vi "GOTOxyz.vi"(6 "reset":bool, 7 "error in (no error)":errorcluster, 9 "Y":dbl format="%#_13g", 10 "X":dbl format="%#_13g") -> (0 "error out":errorcluster)   [LabVIEW 2018]
uses:
  <vilib>/Platform/TimedLoop/XDataNode/timing_clust.ctl
  <vilib>/Platform/TimedLoop/XDataNode/nitl_modes.ctl
  <vilib>/Platform/TimedLoop/XDataNode/wakeup.ctl
  <vilib>/platform/TimedLoop/XDataNode/XDataNode.xnode
  <vilib>/Platform/TimedLoop/XDataNode/XDNodeRunTimeDep.lvlib
  <vilib>/ptbypt/NI_PtbyPt.lvlib
panel:
  out "x*y":dbl
  out "theta":dbl
  in  "Z":dbl format="%#_13g"
  out "T1":dbl
  out "Waveform Chart":dbl(graph)
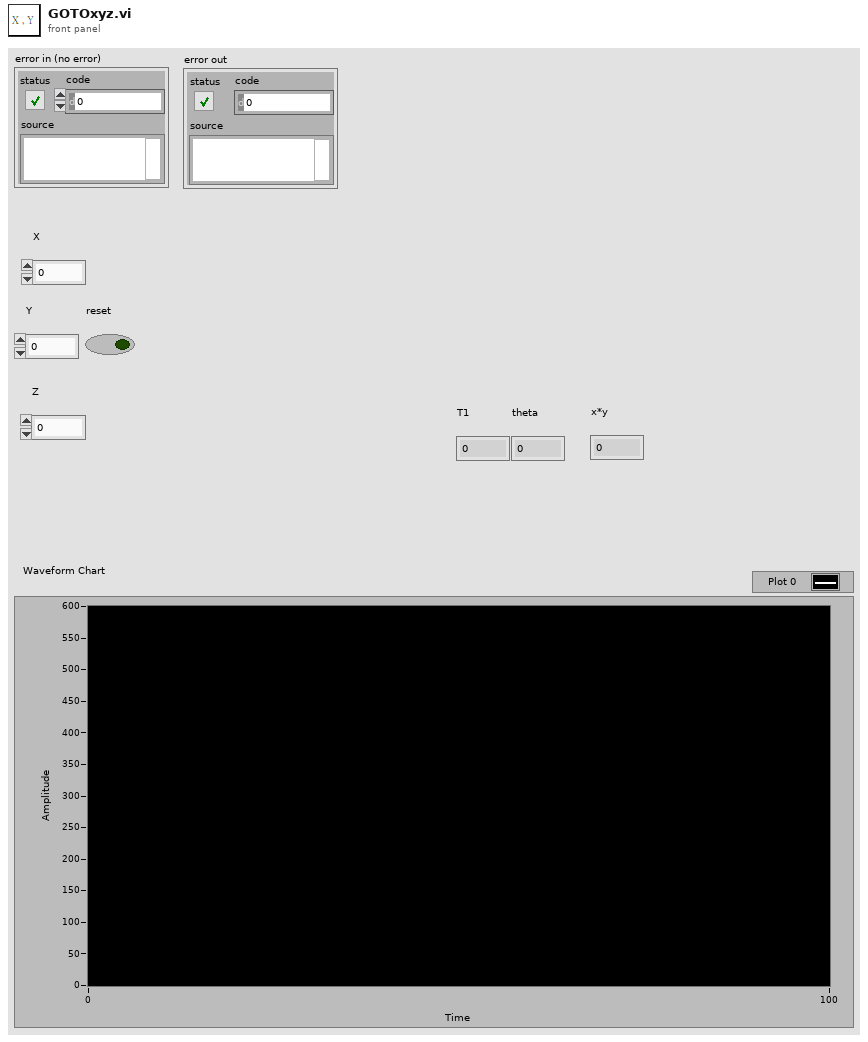
[diagram p1: front panel]
types:
  T1 = typedef "XDNodeRunTimeDep.lvlib/timing_clust.ctl" = cluster{"Expected End [f-1]":u64, "Actual End [f-1]":u64, "Finished Late? [f-1]":bool, "Expected End [i-1]":u64, "Actual End [i-1]":u64, "Finished Late? [i-1]":bool, "Expected Start [i]":u64, "Actual Start [i]":u64, "Expected Start [f]":u64, "Actual Start [f]":u64, "Source Name":string, "Structure Name":string, "Period":i64, "Deadline":i64, "Offset":i64, "Start":i64, "Priority":i32, "Timeout":i32, "Mode":T2, "Wakeup Reason":T3, "Error":errorcluster, "Source Type":string, "Secondary Source Type":string, "Global End Time":u64, "Global Start Time":u64, "Frame Duration":u64, "Iteration Duration":u64, "Assigned CPU":i32, "I/O Scan Engine Mode":u32}
  T2 = typedef "XDNodeRunTimeDep.lvlib/nitl_modes.ctl" = enum32{"No Change", "Process missed periods, maintain original phase", "Discard missed periods, maintain original phase", "Process missed periods, ignore original phase", "Discard missed periods, ignore original phase"}
  T3 = typedef "XDNodeRunTimeDep.lvlib/wakeup.ctl" = enum32{"Normal", "Aborted", "Asynchronous wakeup", "Timing source error", "Timed loop error", "Timeout"}
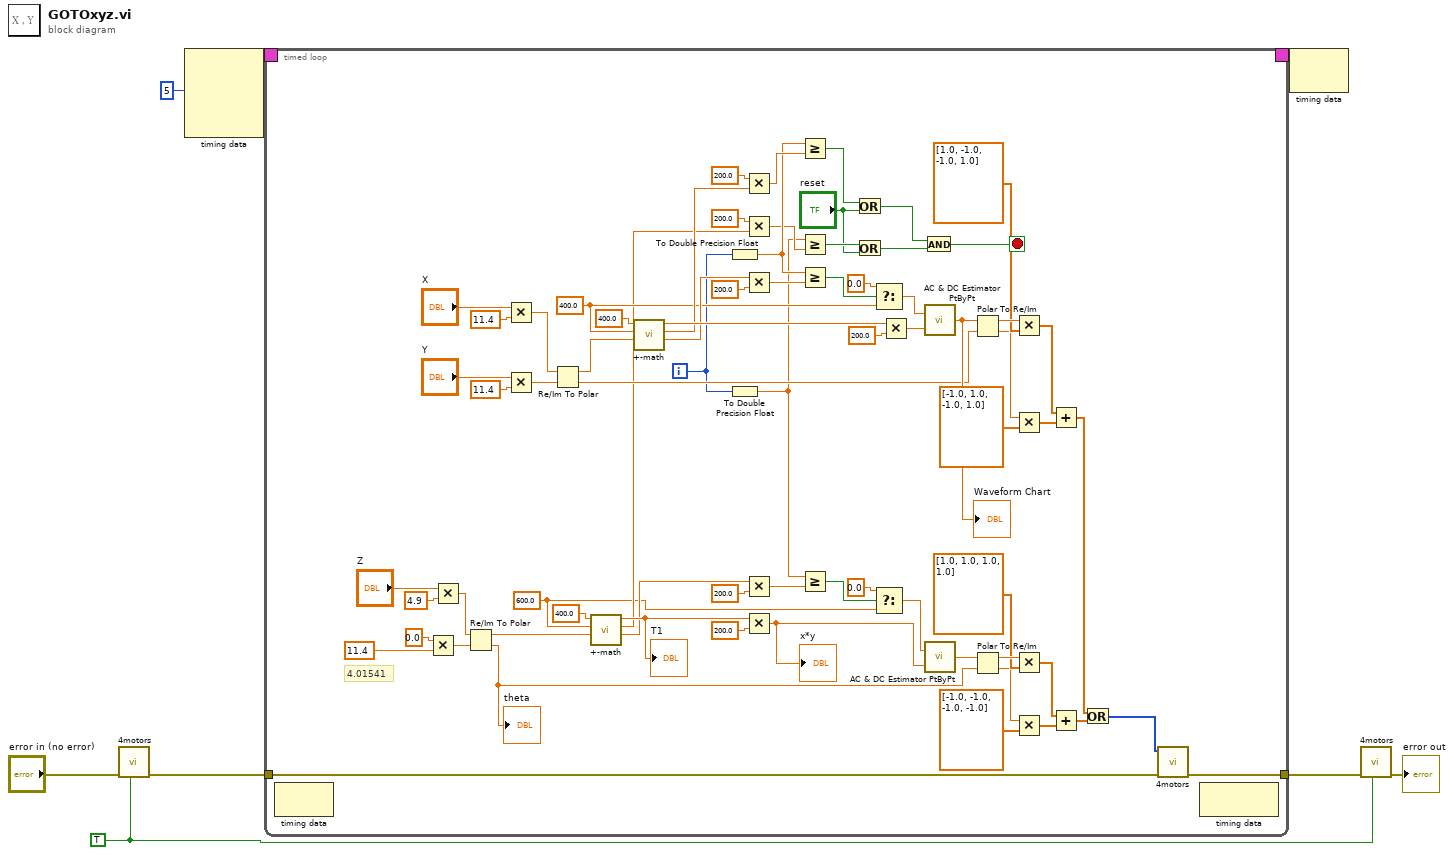
[diagram p0: block diagram]
diagram:
  w3 = TRUE ("Reset")
  n1 = call "4motors.vi"("Reset"=w3, "error in (no error)"="error in (no error)") -> ("error out"=w4:errorcluster)  [unwired: 8 in, 1 out]
  n2 = node-c288(i64 5 ("Period")) -> (w8:T1)  [unwired: 3 in]
  n3 = timed-loop {
    timing: w8 -> [_]
    timing-out: [_] -> w7
    tunnel: [w51] -> w5
    tunnel: w4 -> [w49]
    i -> [w10]
    stop <- w12 stop-if-true
    w18 = 600.0 ("VMAX")
    w50 = 400.0 ("VMAX")
    # "4.01541"
    n4 = node-c288() -> ()  [unwired: 1 in, 1 out]
    n5 = Multiply(x=0.0 ("Y"), y=11.4) -> (x*y=w24:dbl)
    n6 = Multiply(x="Z", y=4.9) -> (x*y=w27:dbl)
    n7 = Re/Im To Polar(2:w24, 3:w27) -> (0:w36:dbl, 1:w38:dbl)
    "theta" <- w36
    n8 = Multiply(x="X", y=11.4) -> (x*y=w60:dbl)
    n9 = Multiply(x="Y", y=11.4) -> (x*y=w57:dbl)
    n10 = Re/Im To Polar(2:w57, 3:w60) -> (0:w69:dbl, 1:w71:dbl)
    n11 = call "+-math.vi"("S"=w38, "VMAX"=w18, "ACC"=400.0) -> ("T2"=w43:dbl, "T3"=w23:dbl, "T1"=w46:dbl)  [unwired: 6 in]
    "T1" <- w46
    n12 = call "+-math.vi"("S"=w71, "VMAX"=w50, "ACC"=400.0) -> ("T2"=w76:dbl, "T3"=w56:dbl, "T1"=w79:dbl)  [unwired: 6 in]
    n13 = To Double Precision Float(number=w10) -> (double precision float=w48:dbl)
    n14 = To Double Precision Float(number=w10) -> (double precision float=w17:dbl)
    n15 = Multiply(x=200.0, y=w56) -> (x*y=w54:dbl)
    n16 = Multiply(x=200.0, y=w23) -> (x*y=w21:dbl)
    n17 = Multiply(x=w76, y=200.0) -> (x*y=w74:dbl)
    n18 = Multiply(x=w43, y=200.0) -> (x*y=w41:dbl)
    n19 = Multiply(x=w46, y=200.0) -> (x*y=w44:dbl)
    "x*y" <- w44
    n20 = Greater Or Equal?(x=w48, y=w54) -> (x >= y?=w53:bool)
    n21 = Greater Or Equal?(x=w17, y=w21) -> (x >= y?=w20:bool)
    n22 = Greater Or Equal?(x=w48, y=w74) -> (x >= y?=w52:bool)
    n23 = Greater Or Equal?(x=w17, y=w41) -> (x >= y?=w19:bool)
    n24 = Or(x=w53, y="reset") -> (x .or. y?=w13:bool)
    n25 = Or(x=w20, y="reset") -> (x .or. y?=w14:bool)
    n26 = Select(t=0.0, s=w52, f=w50) -> (s? t:f=w72:dbl)
    n27 = Select(t=0.0, s=w19, f=w18) -> (s? t:f=w39:dbl)
    n28 = Multiply(x=w79, y=200.0) -> (x*y=w77:dbl)
    n29 = And(x=w13, y=w14) -> (x .and. y?=w12:bool)
    n30 = call <vilib>:"AC & DC Estimator PtByPt.vi"("signal"=w72, "sample length"=w77) -> ("DC estimate (V)"=w70:dbl)  [unwired: 1 in, 2 out]
    "Waveform Chart" <- w70
    n31 = call <vilib>:"AC & DC Estimator PtByPt.vi"("signal"=w39, "sample length"=w44) -> ("DC estimate (V)"=w37:dbl)  [unwired: 1 in, 2 out]
    n32 = Polar To Re/Im(2:w69, 3:w70) -> (0:w66:dbl, 1:w68:dbl)
    n33 = Polar To Re/Im(2:w36, 3:w37) -> (0:w33:dbl, 1:w35:dbl)
    n34 = Multiply(x=w68, y=dbl[] [1.0, -1.0, -1.0, 1.0]) -> (x*y=w64:dbl[])
    n35 = Multiply(x=w66, y=dbl[] [-1.0, 1.0, -1.0, 1.0]) -> (x*y=w63:dbl[])
    n36 = Multiply(x=w35, y=dbl[] [1.0, 1.0, 1.0, 1.0]) -> (x*y=w31:dbl[])
    n37 = Multiply(x=w33, y=dbl[] [-1.0, -1.0, -1.0, -1.0]) -> (x*y=w30:dbl[])
    n38 = Add(x=w64, y=w63) -> (x+y=w16:dbl[])
    n39 = Add(x=w31, y=w30) -> (x+y=w15:dbl[])
    n40 = Or(x=w16, y=w15) -> (x .or. y?=w9:i32[])
    n41 = call "4motors.vi"("error in (no error)"=w49, "Power"=w9) -> ("error out"=w51:errorcluster)  [unwired: 8 in, 1 out]
    n42 = node-c288() -> ()  [unwired: 1 in, 1 out]
  }
  n43 = node-c288(w7) -> ()  [unwired: 1 out]
  n44 = call "4motors.vi"("Reset"=w3, "error in (no error)"=w5) -> ("error out"=→"error out":errorcluster)  [unwired: 8 in, 1 out]
